vi "CmdHeader.vi"(8 "error in (no error)":errorcluster, 9 "TCP/IP Port":i32=3363, 10 "Version":u32=2020, 11 "Project Path":path=path "\\\\vmware-host\\Shared Folders/_Repo/NI-XNET-Monitor-Custom-Device/Source/NI-XNET Monitor Custom Device.lvproj") -> (0 "error out":errorcluster, 3 "Command Out":string)   [LabVIEW 2020, in "Library Builder.lvclass"]
uses:
  Library Builder.lvclass
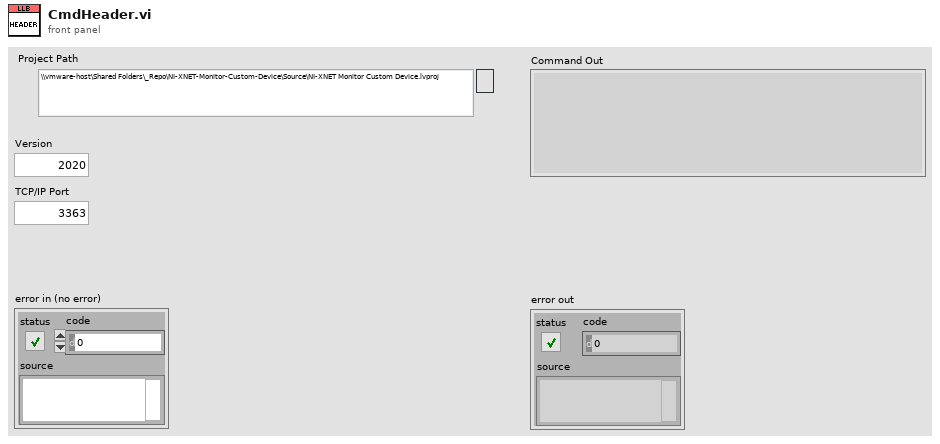
[diagram p1: front panel]
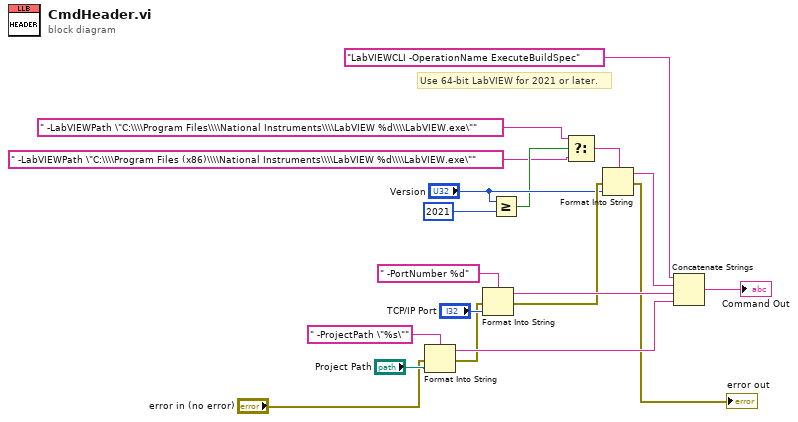
[diagram p0: block diagram]
diagram:
  # "Use 64-bit LabVIEW for 2021 or later."
  n1 = Format Into String(format string=" -ProjectPath \"%s\"", error in="error in (no error)", "Project Path") -> (resulting string=w19:string, error out=w9:errorcluster)  [unwired: 1 in]
  n2 = Format Into String(format string=" -PortNumber %d" ("initial string"), error in=w9, "TCP/IP Port") -> (resulting string=w16:string, error out=w8:errorcluster)  [unwired: 1 in]
  n3 = Greater Or Equal?(x="Version", y=u32 2021 ("Version")) -> (x >= y?=w4:bool)
  n4 = Select(t=" -LabVIEWPath \"C:\\\\Program Files\\\\National Instruments\\\\LabVIEW %d\\\\LabVIEW.exe\"" ("initial string"), s=w4, f=" -LabVIEWPath \"C:\\\\Program Files (x86)\\\\National Instruments\\\\LabVIEW %d\\\\LabVIEW.exe\"" ("initial string")) -> (s? t:f=w3:string)
  n5 = Format Into String(format string=w3, error in=w8, "Version") -> (resulting string=w15:string, error out=→"error out":errorcluster)  [unwired: 1 in]
  n6 = Concatenate Strings("LabVIEWCLI -OperationName ExecuteBuildSpec", w15, w16, w19) -> (→"Command Out":string)
